vi "Live_Camram_Example.vi"() -> ()   [LabVIEW 2019]
doc: "A short program to demonstrate the fundamentals of control and image acquision with the pco.camera series. The program records a sequence of images, with \"live\" updating, until the \"StopRecording\" button is pressed. Use ctrl-H for more help on the individual controls and indicators.\n\nCopyright 2004, 2010 The Cooke Corporation."
uses:
  camera/Camera.lvclass
  pco.sdk/TimingControl/TimingControl.lvlib
  <vilib>/picture/picture.llb/Draw 8-Bit Pixmap.vi
  <vilib>/picture/picture.llb/Draw True-Color Pixmap.vi
panel:
  out "colormap(U8)":u32[](array[numeric])
  in  "Zoom [%]":i32(slide)=26 min=10 max=200 step=5 scale=10.0..200.0
  out "Image":picture
  out "Image(U16)":u16[][](graph)
  in  "Trigger":bool
  in  "data_format":T1(ring)=enum."Mono16"
  out "rawImage":u16[][](array[numeric])
  in  "Image Index":u32 max=1084
  out "Recorded Images":u32
  in  "TriggerMode":T2(ring)
  in  "Quit":bool
  out "Error":errorcluster {"code" format="%x"}
  in  "Stop Record":bool
  out "Recording On":bool
  in  "roiY1":u64=2 min=1 max=1440 step=1
  in  "roiX1":u64=2 min=1 max=1920 step=1
  in  "roiY0":u64=1 max=1439 step=1
  in  "roiX0":u64=1 max=1919 step=1
  out "Image Height":u64
  out "Image Width":u64
  in  "segment":u16=1 min=1 max=4
  in  "Exposure Time [s]":dbl=0.010000000000000002 step=0.001
  # "This example demonstrates recording with live view for cameras with internal memory. \nDuring record, the latest transfered image is shown, after record is stopped, the images insisde the camera's ram can be addressed by index.\nNote that this example will not be fail save, i.e. doesnt react on errors, just handles them forward to the end\n\nUsage:\nSelect your required segment you want to record to, data format and the camera setup before you start the program.\nOnce started, the camera class will be initialized and images will be recorded and displayed automatically\nYou can stop the images by pressing stop record.\nAfter stopped, the image at the selected index will be read from the camera's RAM\nTo finish the program click on quit application, this will force an exit of the camera class\nYou can change your required ROI after and also during the record."
  # "pco.labview"
  # "Camera Setup"
  # "Recording Control"
  # "Parameters for image readout"
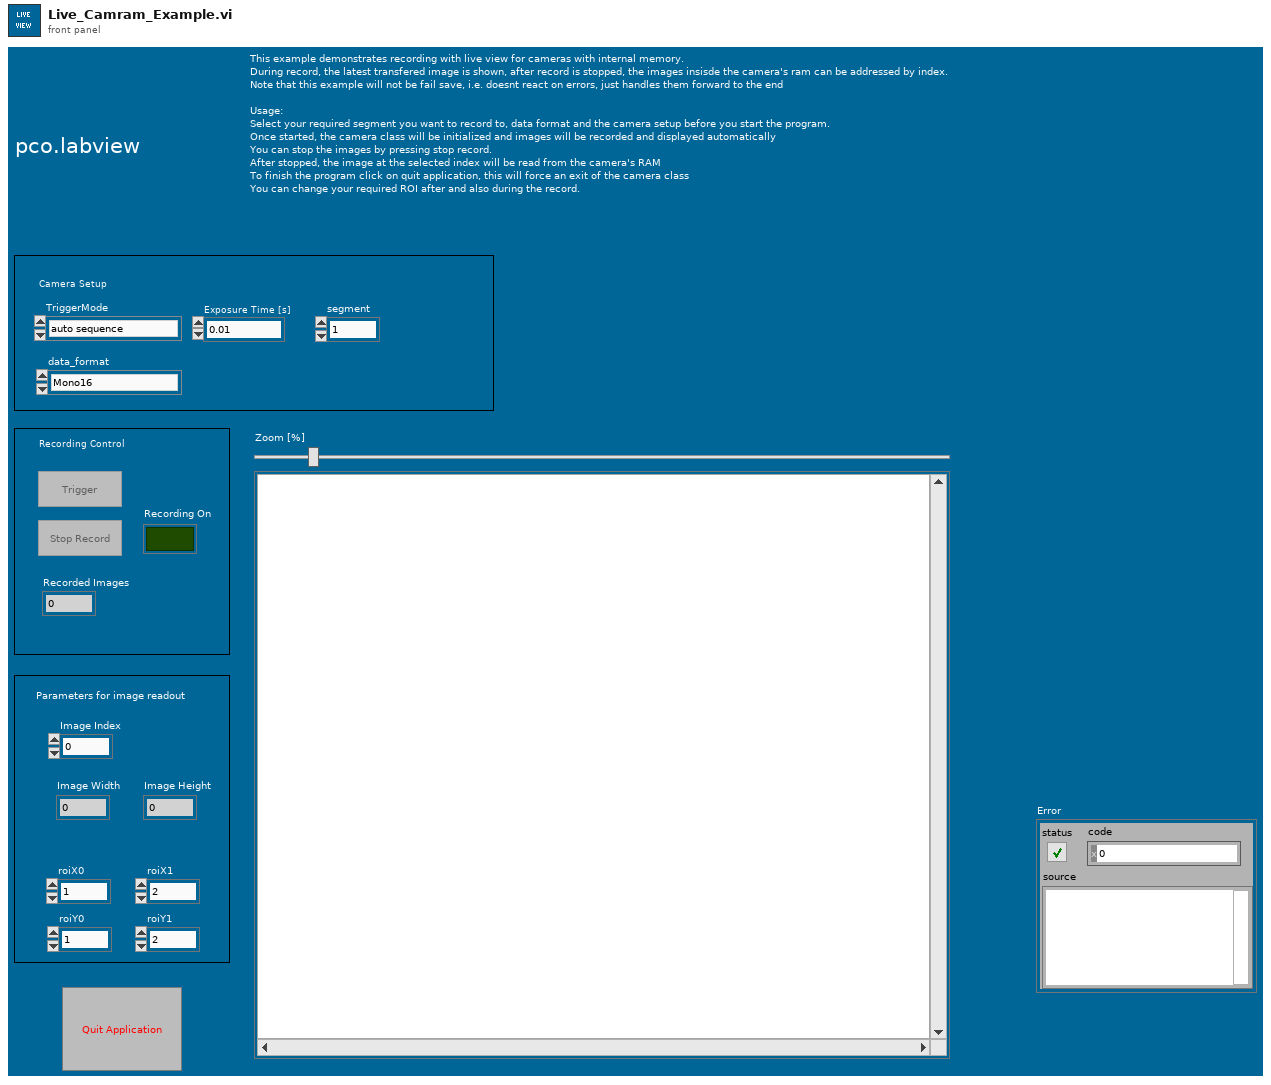
[diagram p1: front panel]
types:
  T1 = enum16{"Undefined", "Mono8", "Mono16", "BGRA8", "RGBA8", "BGRA16", "RGBA16", "CompressedMono8"}
  T2 = enum16{"auto sequence", "software trigger", "external exposure start", "external exposure control"}
  T3 = enum16{"sequence", "sequence non blocking", "ring buffer", "fifo", "tif", "multitif", "pcoraw", "b16", "dicom", "multidicom", "camram_ring", "camram_segment"}
  T4 = enum8{"Enabled", "Disabled", "Disabled and Grayed Out"}
  T5 = cluster{"serial":u32, "type":u16, "sub_type":u16, "interface_type":u16, "bit_resolution":u16, "min_exposure_time_s":dbl, "max_exposure_time_s":dbl, "min_exposure_step_s":dbl, "min_delay_time_s":dbl, "max_delay_time_s":dbl, "min_delay_step_s":dbl, "min_width":u64, "min_height":u64, "max_width":u64, "max_height":u64, "roi_step_horz":u64, "roi_step_vert":u64, "roi_symmetric_horz":bool, "roi_symmetric_vert":bool, "has_timestamp_mode":bool, "has_timestamp_mode_ascii_only":bool, "pixelrate_vec":u32[], "conversion_factor_vec":sgl[], "has_trigger_mode_extexpctrl":bool, "has_acquire_mode":bool, "has_ext_acquire_mode":bool, "has_metadata_mode":bool, "has_ram":bool, "binning_horz_vec":u16[], "binning_vert_vec":u16[], "has_average_binning":bool, "pixel_format_vec":u32[]}
  T6 = cluster{"wSignalNum":u16, "wEnabled":u16, "wType":u16, "wPolarity":u16, "wFilterSetting":u16, "wSelected":u16, "dwParameter":u32[], "dwSignalFunctionality":u32[]}
  T7 = typedef "Camera.lvclass/binning.ctl" = cluster{"vert":u16, "horz":u16, "mode":u16}
  T8 = cluster{"exposure_time_s":dbl, "delay_time_s":dbl, "roi":cluster{"x0":u64, "y0":u64, "x1":u64, "y1":u64}, "timestamp_mode":u16, "pixelrate":u32, "conversion_factor":sgl, "trigger_mode":u16, "acquire_mode":u16, "acquire_sequence_number":u32, "metadata_mode":u16, "noisefilter_mode":u16, "pixel_format":u32, "binning":T7, "auto_exposure":cluster{"region":u16, "min_exposure_s":dbl, "max_exposure_s":dbl}}
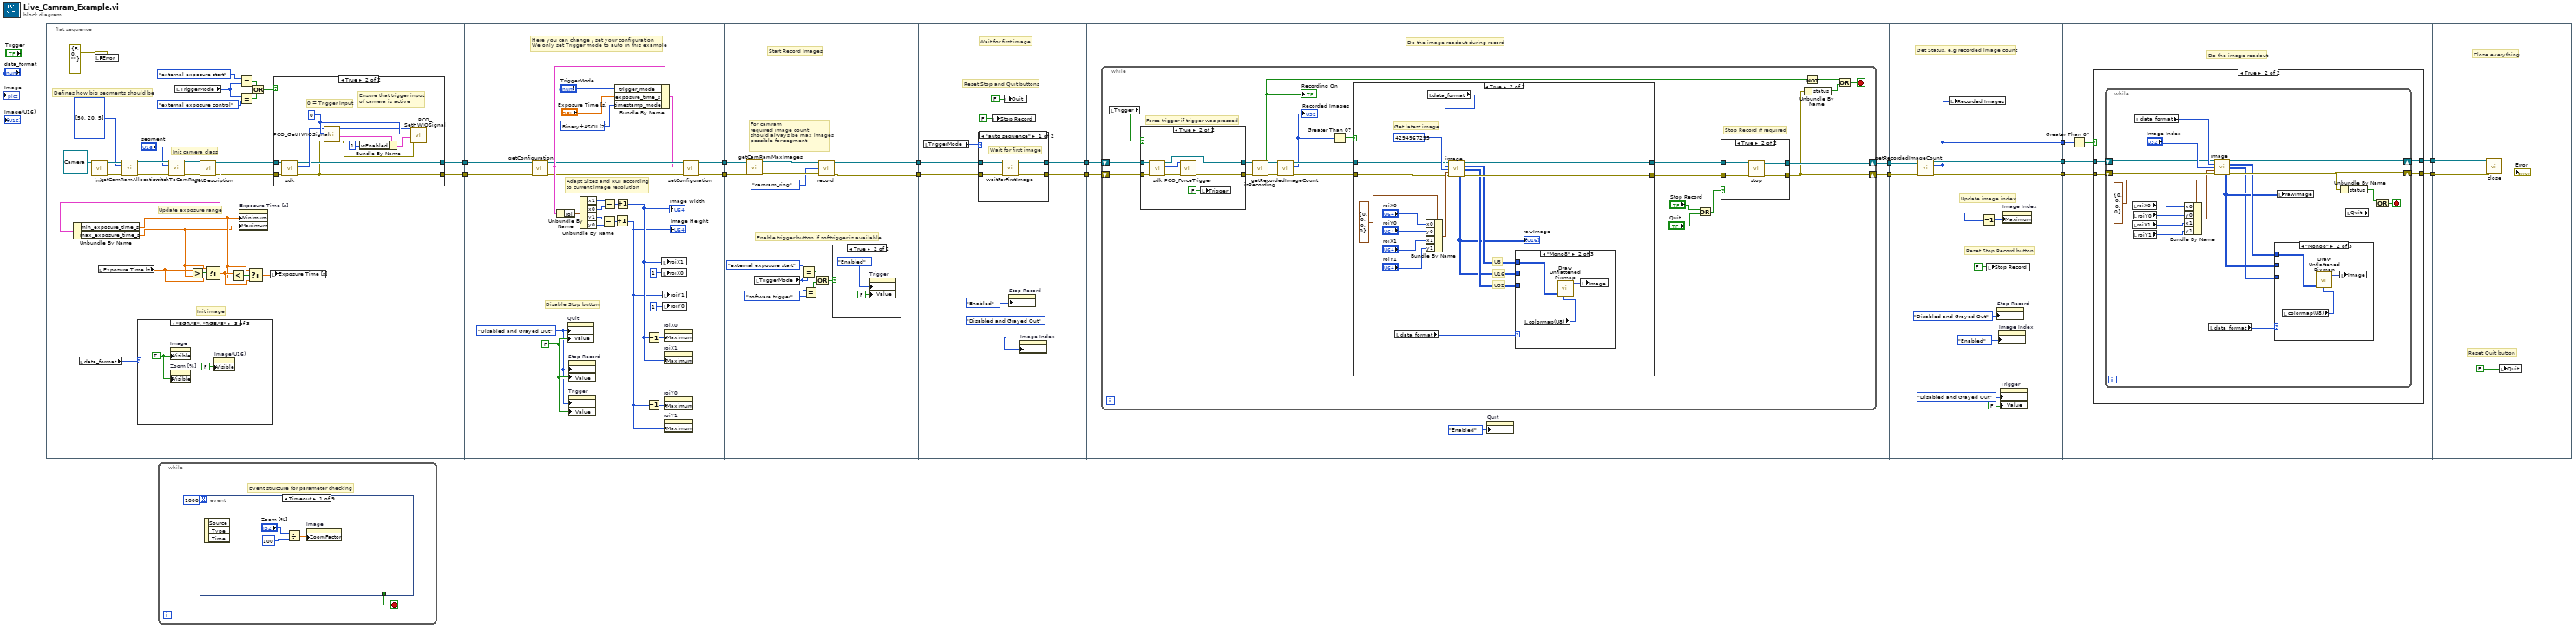
[diagram p0: block diagram]
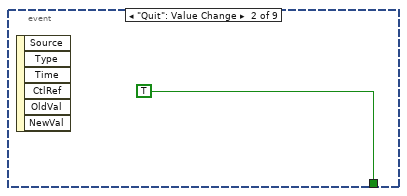
[diagram p2: hidden frame]
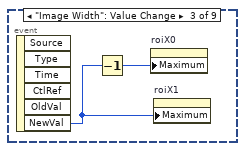
[diagram p3: hidden frame]
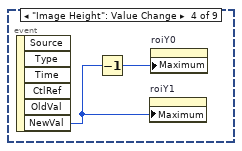
[diagram p4: hidden frame]
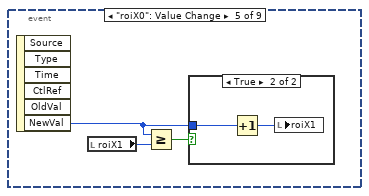
[diagram p5: hidden frame]
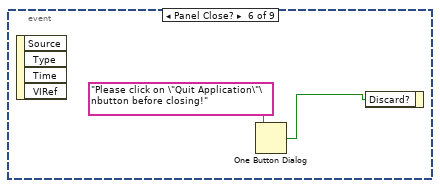
[diagram p7: hidden frame]
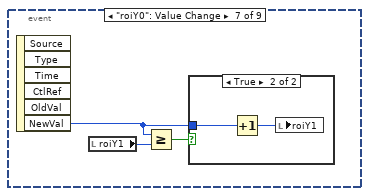
[diagram p8: hidden frame]
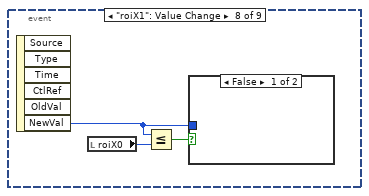
[diagram p10: hidden frame]
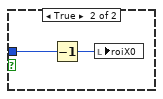
[diagram p11: hidden frame]
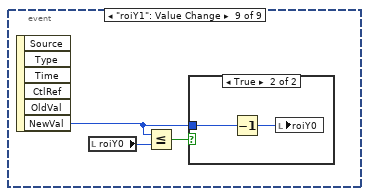
[diagram p12: hidden frame]
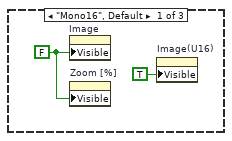
[diagram p15: hidden frame]
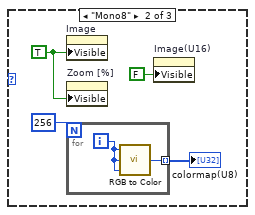
[diagram p16: hidden frame]
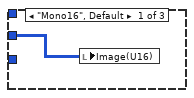
[diagram p20: hidden frame]
diagram:
  n1 = flat-sequence {
    tunnel: [w23] -> w2
    tunnel: [w22] -> w1
    tunnel: [w72] -> w15
    tunnel: [w75] -> w14
    tunnel: w2 -> [w70]
    tunnel: w1 -> [w71]
    tunnel: [w99] -> w9
    tunnel: [w100] -> w8
    tunnel: w14 -> [w97]
    tunnel: w15 -> [w98]
    tunnel: w9 -> [w113]
    tunnel: w8 -> [w114]
    tunnel: [w112] -> w13
    tunnel: [w110] -> w4
    tunnel: w13 -> [w128]
    tunnel: [w126] -> w12
    tunnel: [w125] -> w7
    tunnel: w4 -> [w124]
    tunnel: w12 -> [w198]
    tunnel: [w197] -> w11
    tunnel: w7 -> [w192]
    tunnel: [w191] -> w6
    tunnel: [w190] -> w3
    tunnel: w11 -> [w206]
    tunnel: [w205] -> w10
    tunnel: w6 -> [w204]
    tunnel: [w203] -> w5
    tunnel: w3 -> [w201]
    tunnel: w10 -> [w240]
    tunnel: w5 -> [w238]
    frame #0 {
      # "Defines how big segments should be"
      # "Init image"
      # "Init camera class"
      # "Update exposure range"
      n2 = local read "data_format"() -> (w34:T1)
      n3 = call-dynamic "init.vi"("Camera in"=refnum<class "Camera.lvclass"> refnum) -> ("Camera out"=w31:refnum<class "Camera.lvclass">, "error out"=w30:errorcluster)  [unwired: 8 in]
      n4 = local write "Error"(errorcluster {"status"=FALSE, "code"=0, "source"=""} ("error IO")) -> ()
      n5 = local read "Exposure Time [s]"() -> (w43:dbl)
      n6 = call-dynamic "setCamRamAllocation.vi"("Camera in"=w31, "percents"=u32[] [50, 20, 5], "error in (no error)"=w30) -> ("Camera out"=w33:refnum<class "Camera.lvclass">, "error out"=w32:errorcluster)  [unwired: 11 in]
      n7 = case shown="\"BGRA8\", \"RGBA8\"" w34 {
        frame "Mono16", Default {
          w58 = FALSE ("Visible")
          n8 = property on="Image" class="Pict"("Visible"=w58) -> ()  [unwired: 2 in, 2 out]
          n9 = property on="Zoom [%]" class="Slide (strict)"("Visible"=w58) -> ()  [unwired: 2 in, 2 out]
          n10 = property on="Image(U16)" class="IntGraph (strict)"("Visible"=TRUE) -> ()  [unwired: 2 in, 2 out]
        }
        frame "Mono8" {
          w62 = TRUE ("Visible")
          n11 = property on="Image" class="Pict"("Visible"=w62) -> ()  [unwired: 2 in, 2 out]
          n12 = property on="Zoom [%]" class="Slide (strict)"("Visible"=w62) -> ()  [unwired: 2 in, 2 out]
          n13 = for {
            N: 256 -> [_]
            tunnel: [w64] -> w61 mode=indexing
            i -> [w65]
            n14 = call <vilib>:"RGB to Color.vi"("B"=w65, "G"=w65, "R"=w65) -> ("Color"=w64:u32)
          }
          "colormap(U8)" <- w61
          n15 = property on="Image(U16)" class="IntGraph (strict)"("Visible"=FALSE) -> ()  [unwired: 2 in, 2 out]
        }
        frame "BGRA8", "RGBA8" {
          w66 = TRUE ("Visible")
          n16 = property on="Image" class="Pict"("Visible"=w66) -> ()  [unwired: 2 in, 2 out]
          n17 = property on="Zoom [%]" class="Slide (strict)"("Visible"=w66) -> ()  [unwired: 2 in, 2 out]
          n18 = property on="Image(U16)" class="IntGraph (strict)"("Visible"=FALSE) -> ()  [unwired: 2 in, 2 out]
        }
      }
      n19 = call-dynamic "switchToCamRam.vi"("Camera in"=w33, "segment"="segment", "error in (no error)"=w32) -> ("Camera out"=w28:refnum<class "Camera.lvclass">, "error out"=w27:errorcluster)  [unwired: 11 in]
      n20 = local read "TriggerMode"() -> (w16:T2)
      n21 = call-dynamic "getDescription.vi"("error in (no error)"=w27, "Camera in"=w28) -> ("error out"=w24:errorcluster, "description"=w37:T5, "Camera out"=w25:refnum<class "Camera.lvclass">)  [unwired: 7 in]
      n22 = Unbundle By Name(w37) -> ("min_exposure_time_s"=w36:dbl, "max_exposure_time_s"=w35:dbl)
      n23 = Greater?(x=w43, y=w35) -> (0:w44:bool)
      n24 = Select(t=w35, s=w44, f=w43) -> (s? t:f=w41:dbl)
      n25 = Less?(x=w41, y=w36) -> (x < y?=w42:bool)
      n26 = Equal?(x=T2."external exposure start" ("TriggerMode"), y=w16) -> (x = y?=w20:bool)
      n27 = Equal?(x=w16, y=T2."external exposure control" ("TriggerMode")) -> (x = y?=w19:bool)
      n28 = property on="Exposure Time [s]" class="DigNum (strict)"("Minimum"=w36, "Maximum"=w35) -> ()  [unwired: 2 in, 2 out]
      n29 = Select(t=w36, s=w42, f=w41) -> (s? t:f=w40:dbl)
      n30 = Or(x=w20, y=w19) -> (x .or. y?=w17:bool)
      n31 = local write "Exposure Time [s]"(w40) -> ()
      n32 = case shown="True" w17 {
        tunnel: w25 -> [w46 w50]
        tunnel: w24 -> [w45 w49]
        tunnel: [w45 w47] -> w23
        tunnel: [w46 w48] -> w22
        frame False {
        }
        frame True {
          w55 = u16 0 ("wSignalNum")
          # "0 = Trigger Input"
          # "Ensure that trigger input\nof camera is active"
          n33 = call-dynamic "sdk.vi"("Camera in"=w50, "error in (no error)"=w49) -> ("Camera out"=w48:refnum<class "Camera.lvclass">, "sdk"=w51:u64, "error out"=w47:errorcluster)  [unwired: 11 in]
          n34 = call "PCO_GetHWIOSignal.vi"("error in (no error)"=w47, "wSignalNum"=w55, "ph"=w51) -> ("error out"=w53:errorcluster, "strSignal"=w57:T6, "ph out"=w52:u64)  [unwired: 5 in, 1 out]
          n35 = Bundle By Name(cluster=w57, "wEnabled"=u16 1) -> (w54:T6)
          n36 = call "PCO_SetHWIOSignal.vi"("error in (no error)"=w53, "strSignal"=w54, "wSignalNum"=w55, "ph"=w52) -> ()  [unwired: 5 in, 3 out]
        }
      }
    }
    frame #1 {
      w81 = u16 2 items=["OFF", "Binary", "Binary+ASCII", "ASCII"] ("wTimeStampMode")
      w69 = FALSE ("Stop")
      w68 = T4."Disabled and Grayed Out" ("Disabled")
      # "Disable Stop button"
      # "Adapt Sizes and ROI according\nto current image resolution"
      # "Here you can change / set your configuration\nWe only set Trigger mode to auto in this example"
      n37 = call-dynamic "getConfiguration.vi"("error in (no error)"=w70, "Camera in"=w71) -> ("error out"=w76:errorcluster, "configuration"=w86:T8, "Camera out"=w78:refnum<class "Camera.lvclass">)  [unwired: 7 in]
      n38 = Unbundle By Name(w86) -> ("roi"=w87:cluster{"x0":u64, "y0":u64, "x1":u64, "y1":u64})
      n39 = property on="Quit" class="Bool (strict)"("DisabledEnum"=w68, "Value"=w69) -> ()  [unwired: 2 in, 2 out]
      n40 = property on="Stop Record" class="Bool (strict)"("DisabledEnum"=w68, "Value"=w69) -> ()  [unwired: 2 in, 2 out]
      n41 = property on="Trigger" class="Bool (strict)"("DisabledEnum"=w68, "Value"=w69) -> ()  [unwired: 2 in, 2 out]
      n42 = Unbundle By Name(w87) -> ("x1"=w89:u64, "x0"=w88:u64, "y1"=w91:u64, "y0"=w90:u64)
      n43 = Subtract(x=w91, y=w90) -> (x-y=w93:u64)
      n44 = Subtract(x=w89, y=w88) -> (x-y=w92:u64)
      n45 = Bundle By Name(cluster=w86, "trigger_mode"="TriggerMode", "exposure_time_s"="Exposure Time [s]", "timestamp_mode"=w81) -> (w77:T8)
      n46 = Increment(x=w93) -> (x+1=w73:u64)
      "Image Height" <- w73
      n47 = Increment(x=w92) -> (x+1=w74:u64)
      "Image Width" <- w74
      n48 = Decrement(x=w74) -> (x-1=w84:u64)
      n49 = Decrement(x=w73) -> (x-1=w85:u64)
      n50 = local write "roiX1"(w74) -> ()
      n51 = local write "roiX0"(u64 1 ("roiY0")) -> ()
      n52 = local write "roiY1"(w73) -> ()
      n53 = local write "roiY0"(u64 1 ("roiY0")) -> ()
      n54 = property on="roiX0" class="DigNum (strict)"("Maximum"=w84) -> ()  [unwired: 2 in, 2 out]
      n55 = property on="roiX1" class="DigNum (strict)"("Maximum"=w74) -> ()  [unwired: 2 in, 2 out]
      n56 = property on="roiY0" class="DigNum (strict)"("Maximum"=w85) -> ()  [unwired: 2 in, 2 out]
      n57 = property on="roiY1" class="DigNum (strict)"("Maximum"=w73) -> ()  [unwired: 2 in, 2 out]
      n58 = call-dynamic "setConfiguration.vi"("error in (no error)"=w76, "configuration"=w77, "Camera in"=w78) -> ("error out"=w75:errorcluster, "Camera out"=w72:refnum<class "Camera.lvclass">)  [unwired: 7 in]
    }
    frame #2 {
      # "For camram\nrequired image count \nshould always be max images\npossible for segment"
      # "Enable trigger button if softtrigger is available"
      # "Start Record Images"
      n59 = call-dynamic "getCamRamMaxImages.vi"("Camera in"=w98, "error in (no error)"=w97) -> ("Camera out"=w95:refnum<class "Camera.lvclass">, "error out"=w96:errorcluster)  [unwired: 11 in, 1 out]
      n60 = local read "TriggerMode"() -> (w105:T2)
      n61 = Equal?(x=T2."external exposure start" ("TriggerMode"), y=w105) -> (x = y?=w102:bool)
      n62 = Equal?(x=w105, y=T2."software trigger" ("TriggerMode")) -> (x = y?=w101:bool)
      n63 = Or(x=w102, y=w101) -> (x .or. y?=w103:bool)
      n64 = call-dynamic "record.vi"("Camera in"=w95, "record_mode"=T3."camram_ring", "error in (no error)"=w96) -> ("Camera out"=w100:refnum<class "Camera.lvclass">, "error out"=w99:errorcluster)  [unwired: 11 in]
      n65 = case shown="True" w103 {
        frame False {
        }
        frame True {
          n66 = property on="Trigger" class="Bool (strict)"("DisabledEnum"=T4."Enabled" ("Disabled"), "Value"=FALSE ("Trigger")) -> ()  [unwired: 2 in, 2 out]
        }
      }
    }
    frame #3 {
      # "Wait for first image"
      # "Reset Stop and Quit buttons"
      n67 = local read "TriggerMode"() -> (w109:T2)
      n68 = case shown="\"auto sequence\"" w109 {
        tunnel: w114 -> [w121 w123]
        tunnel: w113 -> [w120 w122]
        tunnel: [w119 w122] -> w112
        tunnel: [w118 w123] -> w110
        frame "auto sequence" {
          # "Wait for first image"
          n69 = call-dynamic "waitForFirstImage.vi"("error in (no error)"=w120, "Camera in"=w121) -> ("error out"=w119:errorcluster, "Camera out"=w118:refnum<class "Camera.lvclass">)  [unwired: 8 in]
        }
        frame Default {
        }
      }
      n70 = local write "Stop Record"(FALSE ("Stop Record")) -> ()
      n71 = local write "Quit"(FALSE ("Stop")) -> ()
      n72 = property on="Stop Record" class="Bool (strict)"("DisabledEnum"=T4."Enabled" ("Disabled")) -> ()  [unwired: 2 in, 2 out]
      n73 = property on="Image Index" class="DigNum (strict)"("DisabledEnum"=T4."Disabled and Grayed Out" ("Disabled")) -> ()  [unwired: 2 in, 2 out]
    }
    frame #4 {
      # "Do the image readout during record"
      n74 = while {
        shift-right: [w131] -> w126
        shift-left: w128 -> [w135]
        shift-right: [w132] -> w125
        shift-left: w124 -> [w136]
        stop <- w147 stop-if-true
        # "Force trigger if trigger was pressed"
        # "Stop Record if required"
        n75 = local read "Trigger"() -> (w137:bool)
        n76 = case shown="True" w137 {
          tunnel: w136 -> [w176 w181]
          tunnel: w135 -> [w175 w180]
          tunnel: [w176 w179] -> w134
          tunnel: [w175 w178] -> w133
          frame False {
          }
          frame True {
            n77 = call-dynamic "sdk.vi"("Camera in"=w181, "error in (no error)"=w180) -> ("Camera out"=w179:refnum<class "Camera.lvclass">, "sdk"=w182:u64, "error out"=w183:errorcluster)  [unwired: 11 in]
            n78 = call "PCO_ForceTrigger.vi"("error in (no error)"=w183, "ph"=w182) -> ("error out"=w178:errorcluster)  [unwired: 6 in, 3 out]
            n79 = local write "Trigger"(FALSE ("Trigger")) -> ()
          }
        }
        n80 = call-dynamic "isRecording.vi"("Camera in"=w134, "error in (no error)"=w133) -> ("Camera out"=w142:refnum<class "Camera.lvclass">, "recording"=w145:bool, "error out"=w141:errorcluster)  [unwired: 11 in]
        "Recording On" <- w145
        n81 = call-dynamic "getRecordedImageCount.vi"("Camera in"=w142, "error in (no error)"=w141) -> ("Camera out"=w139:refnum<class "Camera.lvclass">, "recorded_image_count"=w129:u32, "error out"=w140:errorcluster)  [unwired: 11 in]
        "Recorded Images" <- w129
        n82 = Greater Than 0?(x=w129) -> (x > 0?=w130:bool)
        n83 = case shown="True" w130 {
          tunnel: [w151 w163] -> w143
          tunnel: w140 -> [w151 w160]
          tunnel: w139 -> [w152 w154]
          tunnel: [w152 w153] -> w138
          frame False {
          }
          frame True {
            # "U32"
            # "U8"
            # "U16"
            # "Get latest image"
            n84 = local read "data_format"() -> (w155:T1)
            n85 = Bundle By Name(cluster=cluster{"x0":u64, "y0":u64, "x1":u64, "y1":u64} {"x0"=0, "y0"=0, "x1"=0, "y1"=0} ("roi"), "x0"="roiX0", "y0"="roiY0", "x1"="roiX1", "y1"="roiY1") -> (w164:cluster{"x0":u64, "y0":u64, "x1":u64, "y1":u64})
            n86 = local read "data_format"() -> (w159:T1)
            n87 = call-dynamic "image.vi"("Camera in"=w154, "data_format"=w159, "image_index"=u32 4294967295 ("dwImgIdx"), "crop"=w164, "error in (no error)"=w160) -> ("Camera out"=w153:refnum<class "Camera.lvclass">, "image (U8)"=w157:u8[][], "image (U32)"=w158:u32[][], "raw_image (U16)"=w156:u16[][], "error out"=w163:errorcluster)  [unwired: 2 in, 4 out]
            "rawImage" <- w156
            n88 = case shown="\"Mono8\"" w155 {
              tunnel: w158 -> [_ _ w174]
              tunnel: w157 -> [_ w172 _]
              tunnel: w156 -> [w169 _ _]
              frame "Mono16", Default {
                n89 = local write "Image(U16)"(w169) -> ()
              }
              frame "Mono8" {
                n90 = local read "colormap(U8)"() -> (w171:u32[])
                n91 = call-poly <vilib>:"Draw Unflattened Pixmap.vi"("data"=w172, "color table"=w171) -> ("new picture"=w170:picture)  [unwired: 7 in]
                n92 = local write "Image"(w170) -> ()
              }
              frame "BGRA8", "RGBA8" {
                n93 = call-poly <vilib>:"Draw Unflattened Pixmap.vi"("data (RGB format)"=w174) -> ("new picture"=w173:picture)  [unwired: 8 in]
                n94 = local write "Image"(w173) -> ()
              }
            }
          }
        }
        n95 = Or(x="Stop Record", y="Quit") -> (x .or. y?=w148:bool)
        n96 = case shown="True" w148 {
          tunnel: w143 -> [w185 w186]
          tunnel: [w184 w188] -> w132
          tunnel: [w185 w189] -> w131
          tunnel: w138 -> [w184 w187]
          frame False {
          }
          frame True {
            n97 = call-dynamic "stop.vi"("error in (no error)"=w186, "Camera in"=w187) -> ("error out"=w189:errorcluster, "Camera out"=w188:refnum<class "Camera.lvclass">)  [unwired: 8 in]
          }
        }
        n98 = Unbundle By Name(w131) -> ("status"=w146:bool)
        n99 = Not(x=w145) -> (.not. x?=w144:bool)
        n100 = Or(x=w144, y=w146) -> (x .or. y?=w147:bool)
      }
      n101 = property on="Quit" class="Bool (strict)"("DisabledEnum"=T4."Enabled" ("Disabled")) -> ()  [unwired: 2 in, 2 out]
    }
    frame #5 {
      # "Update image index"
      # "Reset Stop Record button"
      # "Get Status, e.g recorded image count"
      n102 = call-dynamic "getRecordedImageCount.vi"("Camera in"=w192, "error in (no error)"=w198) -> ("Camera out"=w191:refnum<class "Camera.lvclass">, "recorded_image_count"=w190:u32, "error out"=w197:errorcluster)  [unwired: 11 in]
      n103 = local write "Recorded Images"(w190) -> ()
      n104 = Decrement(x=w190) -> (x-1=w195:u32)
      n105 = local write "Stop Record"(FALSE ("Stop Record")) -> ()
      n106 = property on="Stop Record" class="Bool (strict)"("DisabledEnum"=T4."Disabled and Grayed Out" ("Disabled")) -> ()  [unwired: 2 in, 2 out]
      n107 = property on="Image Index" class="DigNum (strict)"("DisabledEnum"=T4."Enabled" ("Disabled")) -> ()  [unwired: 2 in, 2 out]
      n108 = property on="Trigger" class="Bool (strict)"("DisabledEnum"=T4."Disabled and Grayed Out" ("Disabled"), "Value"=FALSE ("Trigger")) -> ()  [unwired: 2 in, 2 out]
      n109 = property on="Image Index" class="DigNum (strict)"("Maximum"=w195) -> ()  [unwired: 2 in, 2 out]
    }
    frame #6 {
      # "Do the image readout"
      n110 = Greater Than 0?(x=w201) -> (x > 0?=w202:bool)
      n111 = case shown="True" w202 {
        tunnel: w206 -> [w207 w212]
        tunnel: [w207 w211] -> w205
        tunnel: w204 -> [w208 w210]
        tunnel: [w208 w209] -> w203
        frame False {
        }
        frame True {
          n112 = while {
            shift-right: [w223] -> w211
            shift-left: w212 -> [w231]
            shift-right: [w217] -> w209
            shift-left: w210 -> [w218]
            stop <- w225 stop-if-true
            n113 = local read "roiX0"() -> (w221:u64)
            n114 = local read "roiX1"() -> (w229:u64)
            n115 = local read "roiY0"() -> (w222:u64)
            n116 = local read "roiY1"() -> (w228:u64)
            n117 = local read "data_format"() -> (w219:T1)
            n118 = Bundle By Name(cluster=cluster{"x0":u64, "y0":u64, "x1":u64, "y1":u64} {"x0"=0, "y0"=0, "x1"=0, "y1"=0} ("roi"), "x0"=w221, "y0"=w222, "x1"=w229, "y1"=w228) -> (w230:cluster{"x0":u64, "y0":u64, "x1":u64, "y1":u64})
            n119 = local read "data_format"() -> (w216:T1)
            n120 = call-dynamic "image.vi"("Camera in"=w218, "data_format"=w219, "image_index"="Image Index", "crop"=w230, "error in (no error)"=w231) -> ("Camera out"=w217:refnum<class "Camera.lvclass">, "image (U8)"=w215:u8[][], "image (U32)"=w213:u32[][], "raw_image (U16)"=w214:u16[][], "error out"=w223:errorcluster)  [unwired: 2 in, 4 out]
            n121 = case shown="\"Mono8\"" w216 {
              tunnel: w213 -> [_ _ w237]
              tunnel: w215 -> [_ w235 _]
              tunnel: w214 -> [w232 _ _]
              frame "Mono16", Default {
                n122 = local write "Image(U16)"(w232) -> ()
              }
              frame "Mono8" {
                n123 = local read "colormap(U8)"() -> (w234:u32[])
                n124 = call-poly <vilib>:"Draw Unflattened Pixmap.vi"("data"=w235, "color table"=w234) -> ("new picture"=w233:picture)  [unwired: 7 in]
                n125 = local write "Image"(w233) -> ()
              }
              frame "BGRA8", "RGBA8" {
                n126 = call-poly <vilib>:"Draw Unflattened Pixmap.vi"("data (RGB format)"=w237) -> ("new picture"=w236:picture)  [unwired: 8 in]
                n127 = local write "Image"(w236) -> ()
              }
            }
            n128 = local write "rawImage"(w214) -> ()
            n129 = Unbundle By Name(w223) -> ("status"=w226:bool)
            n130 = local read "Quit"() -> (w227:bool)
            n131 = Or(x=w226, y=w227) -> (x .or. y?=w225:bool)
          }
        }
      }
    }
    frame #7 {
      # "Close everything"
      # "Reset Quit button"
      n132 = call-dynamic "close.vi"("error in (no error)"=w240, "Camera in"=w238) -> ("error out"=→"Error":errorcluster)  [unwired: 9 in]
      n133 = local write "Quit"(FALSE ("Stop Record")) -> ()
    }
  }
  n134 = while {
    stop <- w242 stop-if-true
    # "Event structure for parameter checking"
    n135 = event shown="[0] Timeout" {
      selector: _ -> [_ _ _ _ _ _ _ _ _]
      dyn-events: _ -> [_ _ _ _ _ _ _ _ _]
      timeout: 1000 -> [_ _ _ _ _ _ _ _ _]
      tunnel: [_ TRUE _ _ _ _ _ _ _] -> w242
      event Timeout {
        n136 = event-data() -> ()  [unwired: 1 in, 3 out]
        n137 = Divide(x="Zoom [%]", y=100 ("Zoom [%]")) -> (x/y=w245:dbl)
        n138 = property on="Image" class="Pict"("ZoomFactor"=w245) -> ()  [unwired: 2 in, 2 out]
      }
      event "Quit": Value Change {
        n139 = event-data() -> ()  [unwired: 1 in, 6 out]
      }
      event "Image Width": Value Change {
        n140 = event-data() -> ("NewVal"=w248:u64)  [unwired: 1 in, 5 out]
        n141 = Decrement(x=w248) -> (x-1=w249:u64)
        n142 = property on="roiX0" class="DigNum (strict)"("Maximum"=w249) -> ()  [unwired: 2 in, 2 out]
        n143 = property on="roiX1" class="DigNum (strict)"("Maximum"=w248) -> ()  [unwired: 2 in, 2 out]
      }
      event "Image Height": Value Change {
        n144 = event-data() -> ("NewVal"=w250:u64)  [unwired: 1 in, 5 out]
        n145 = Decrement(x=w250) -> (x-1=w251:u64)
        n146 = property on="roiY1" class="DigNum (strict)"("Maximum"=w250) -> ()  [unwired: 2 in, 2 out]
        n147 = property on="roiY0" class="DigNum (strict)"("Maximum"=w251) -> ()  [unwired: 2 in, 2 out]
      }
      event "roiX0": Value Change {
        n148 = event-data() -> ("NewVal"=w252:u64)  [unwired: 1 in, 5 out]
        n149 = local read "roiX1"() -> (w254:u64)
        n150 = Greater Or Equal?(x=w252, y=w254) -> (x >= y?=w253:bool)
        n151 = case shown="True" w253 {
          tunnel: w252 -> [_ w256]
          frame False {
          }
          frame True {
            n152 = Increment(x=w256) -> (x+1=w255:u64)
            n153 = local write "roiX1"(w255) -> ()
          }
        }
      }
      event Panel Close? {
        n154 = event-data() -> ()  [unwired: 1 in, 4 out]
        n155 = One Button Dialog(message="Please click on \"Quit Application\"\nbutton before closing!") -> (true=w257:bool)  [unwired: 1 in]
        n156 = event-data("Discard?"=w257) -> ()  [unwired: 1 in, 1 out]
      }
      event "roiY0": Value Change {
        n157 = event-data() -> ("NewVal"=w259:u64)  [unwired: 1 in, 5 out]
        n158 = local read "roiY1"() -> (w261:u64)
        n159 = Greater Or Equal?(x=w259, y=w261) -> (x >= y?=w260:bool)
        n160 = case shown="True" w260 {
          tunnel: w259 -> [_ w263]
          frame False {
          }
          frame True {
            n161 = Increment(x=w263) -> (x+1=w262:u64)
            n162 = local write "roiY1"(w262) -> ()
          }
        }
      }
      event "roiX1": Value Change {
        n163 = event-data() -> ("NewVal"=w264:u64)  [unwired: 1 in, 5 out]
        n164 = local read "roiX0"() -> (w266:u64)
        n165 = Less Or Equal?(x=w264, y=w266) -> (x <= y?=w265:bool)
        n166 = case shown="False" w265 {
          tunnel: w264 -> [_ w268]
          frame False {
          }
          frame True {
            n167 = Decrement(x=w268) -> (x-1=w267:u64)
            n168 = local write "roiX0"(w267) -> ()
          }
        }
      }
      event "roiY1": Value Change {
        n169 = event-data() -> ("NewVal"=w269:u64)  [unwired: 1 in, 5 out]
        n170 = local read "roiY0"() -> (w271:u64)
        n171 = Less Or Equal?(x=w269, y=w271) -> (x <= y?=w270:bool)
        n172 = case shown="True" w270 {
          tunnel: w269 -> [_ w273]
          frame False {
          }
          frame True {
            n173 = Decrement(x=w273) -> (x-1=w272:u64)
            n174 = local write "roiY0"(w272) -> ()
          }
        }
      }
    }
  }
